vi "Point Value Map EXAMPLE.vi"() -> ()   [LabVIEW 2017]
uses:
  <vilib>/addons/PointValueMap/controls/Point.ctl
  <vilib>/addons/PointValueMap/controls/DataTypes.ctl
  <vilib>/addons/PointValueMap/PointValueMap.lvlib
panel:
  out "Map Content Point - Originals":T1[](array[typedef])
  out "Map Content Points - Copies":T1[](array[typedef])
  out "Map Content Names - Copies":string[](array[string])
  out "Map Content Names - Originals":string[](array[string])
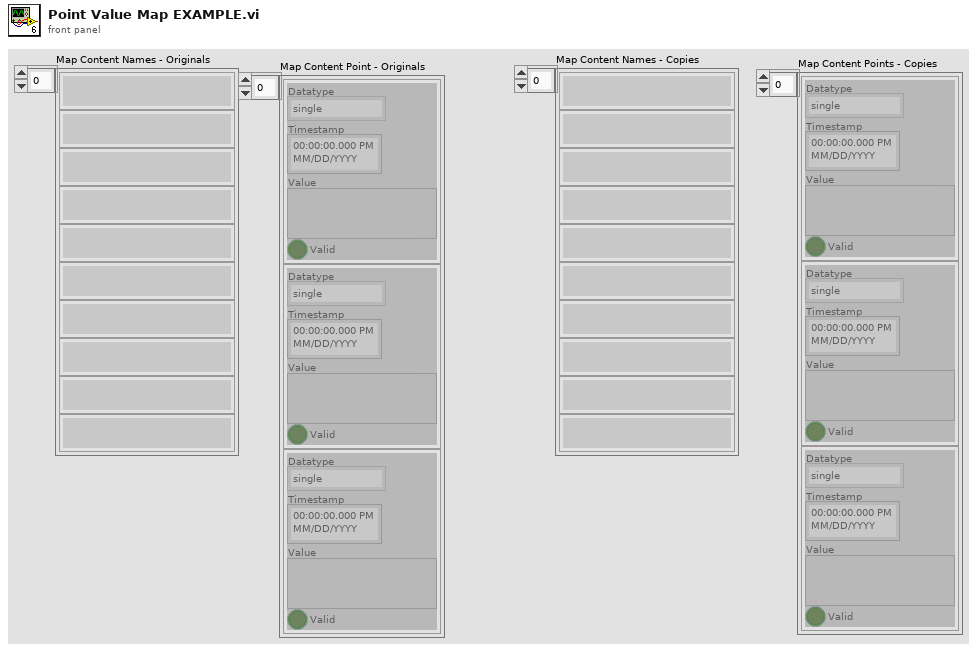
[diagram p1: front panel]
types:
  T1 = typedef "PointValueMap.lvlib/Point.ctl" = cluster{"Datatype":T2, "Timestamp":timestamp, "Value":variant, "Valid":bool}
  T2 = typedef "PointValueMap.lvlib/DataTypes.ctl" = enum16{"single", "double", "i32", "string", "variant"}
  T3 = typedef "PointValueMap.lvlib/PointMap.ctl" = refnum<data-value>
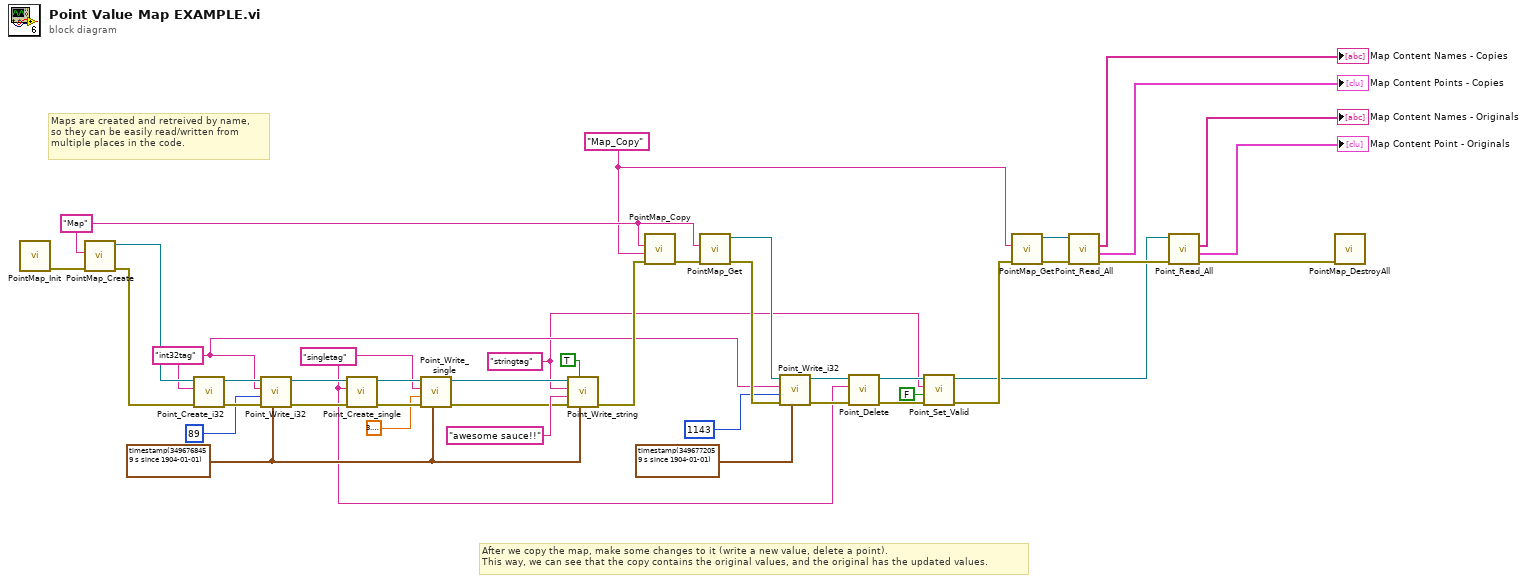
[diagram p0: block diagram]
diagram:
  w20 = "Map_Copy" ("New Map Name")
  w4 = "stringtag" ("Tag")
  w9 = "singletag" ("Tag")
  w33 = timestamp(3496768459.468086 s since 1904-01-01) ("Time Stamp")
  w8 = "int32tag" ("Tag")
  w21 = "Map" ("Name")
  # "Maps are created and retreived by name, \nso they can be easily read/written from \nmultiple places in the code."
  # "After we copy the map, make some changes to it (write a new value, delete a point).\nThis way, we can see that the copy contains the original values, and the original has the updated values."
  n1 = call <vilib>:"PointMap_Init.vi"() -> ("error out"=w42:errorcluster)  [unwired: 11 in]
  n2 = call <vilib>:"PointMap_Create.vi"("error in (no error)"=w42, "Name"=w21) -> ("error out"=w16:errorcluster, "Map Out"=w17:T3)  [unwired: 8 in]
  n3 = call <vilib>:"Point_Create_i32.vi"("Error In"=w16, "Tag"=w8, "Map"=w17) -> ("Error Out"=w40:errorcluster, "Map Out"=w41:T3)  [unwired: 7 in]
  n4 = call <vilib>:"Point_Write_i32.vi"("Time Stamp"=w33, "Error In"=w40, "Value"=89, "Tag"=w8, "Map"=w41) -> ("Error Out"=w37:errorcluster, "Map Out"=w39:T3)  [unwired: 5 in]
  n5 = call <vilib>:"Point_Create_single.vi"("Error In"=w37, "Tag"=w9, "Map"=w39) -> ("Error Out"=w35:errorcluster, "Map Out"=w36:T3)  [unwired: 7 in]
  n6 = call <vilib>:"Point_Write_single.vi"("Time Stamp"=w33, "Error In"=w35, "Value"=sgl 3.1415927, "Tag"=w9, "Map"=w36) -> ("Error Out"=w14:errorcluster, "Map Out"=w15:T3)  [unwired: 5 in]
  n7 = call <vilib>:"Point_Write_string.vi"("Time Stamp"=w33, "Auto Create?"=TRUE, "Error In"=w14, "Value"="awesome sauce!!", "Tag"=w4, "Map"=w15) -> ("Error Out"=w31:errorcluster)  [unwired: 4 in, 1 out]
  n8 = call <vilib>:"PointMap_Copy.vi"("error in (no error)"=w31, "Destination Map Name"=w20, "Source Map Name"=w21) -> ("error out"=w30:errorcluster)  [unwired: 8 in]
  n9 = call <vilib>:"PointMap_Get.vi"("error in (no error)"=w30, "Name"=w21) -> ("error out"=w28:errorcluster, "Map Out"=w27:T3)  [unwired: 7 in, 1 out]
  n10 = call <vilib>:"Point_Write_i32.vi"("Time Stamp"=timestamp(3496772059.468 s since 1904-01-01), "Error In"=w28, "Value"=1143, "Tag"=w8, "Map"=w27) -> ("Error Out"=w18:errorcluster, "Map Out"=w19:T3)  [unwired: 5 in]
  n11 = call <vilib>:"Point_Delete.vi"("Error In"=w18, "Tag"=w9, "Map"=w19) -> ("Error Out"=w6:errorcluster, "Map Out"=w7:T3)  [unwired: 7 in]
  n12 = call <vilib>:"Point_Set_Valid.vi"("Error In"=w6, "Valid?"=FALSE, "Tag"=w4, "Map"=w7) -> ("Error Out"=w5:errorcluster, "Map Out"=w2:T3)  [unwired: 6 in]
  n13 = call <vilib>:"PointMap_Get.vi"("error in (no error)"=w5, "Name"=w20) -> ("error out"=w24:errorcluster, "Map Out"=w25:T3)  [unwired: 7 in, 1 out]
  n14 = call <vilib>:"Point_Read_All.vi"("Error In"=w24, "Map"=w25) -> ("Error Out"=w23:errorcluster, "Points"=→"Map Content Points - Copies":T1[], "Names"=→"Map Content Names - Copies":string[])  [unwired: 6 in, 1 out]
  n15 = call <vilib>:"Point_Read_All.vi"("Error In"=w23, "Map"=w2) -> ("Error Out"=w12:errorcluster, "Points"=→"Map Content Point - Originals":T1[], "Names"=→"Map Content Names - Originals":string[])  [unwired: 6 in, 1 out]
  n16 = call <vilib>:"PointMap_DestroyAll.vi"("error in (no error)"=w12) -> ()  [unwired: 10 in, 1 out]
